vi "Sub Pic Write Data.vi"(8 "error in (no error)":errorcluster, 10 "data (RGB format)":u32[][](array[numeric]) format="%x", 11 "Main Panel in":refnum<class "Main Panel.lvclass">) -> (0 "error out":errorcluster, 3 "Main Panel out":refnum<class "Main Panel.lvclass">)   [LabVIEW 2018, in "Main Panel.lvlib" / "Main Panel.lvclass"]
uses:
  Main Panel.lvclass
  Main Panel.lvclass/Main Panel.ctl
  <vilib>/picture/picture.llb/Draw True-Color Pixmap.vi
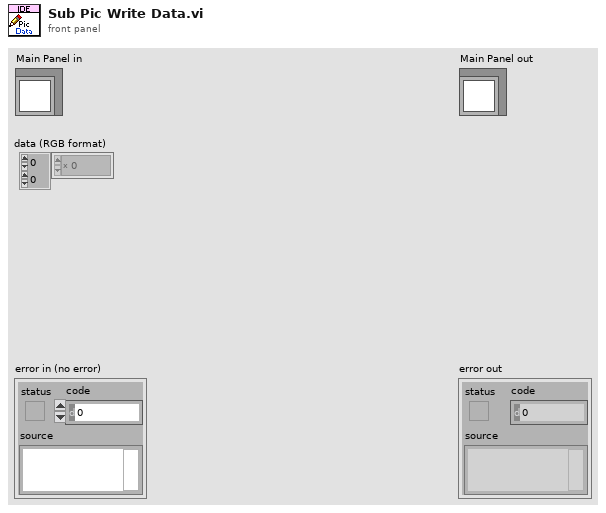
[diagram p1: front panel]
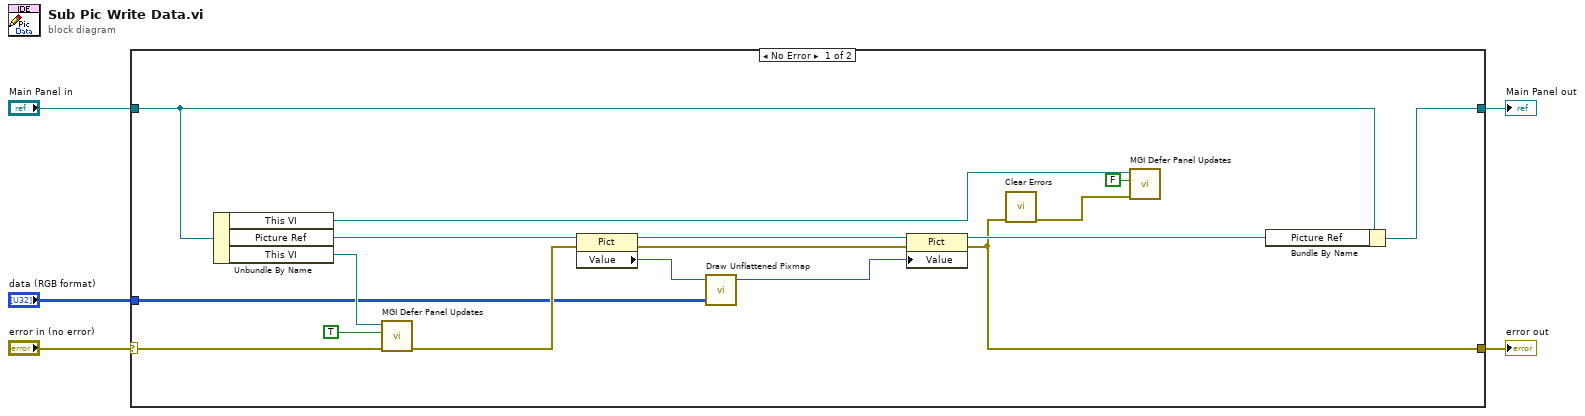
[diagram p0: block diagram]
diagram:
  n1 = case shown="No Error" "error in (no error)" {
    selector: "error in (no error)" -> [w20 w24]
    tunnel: [w6 w24] -> w4
    tunnel: [w11 w23] -> w2
    tunnel: "Main Panel in" -> [w22 w23]
    tunnel: "data (RGB format)" -> [w12 _]
    frame No Error {
      n2 = Unbundle By Name(w22) -> ("This VI"=w8:refnum<vi>, "Picture Ref"=w18:refnum<vi>, "This VI"=w21:refnum<vi>)
      n3 = call <userlib>:"MGI Defer Panel Updates.vi"("Error In"=w20, "Defer Updates?"=TRUE, "VI Reference (Caller)"=w21) -> ("Error Out"=w17:errorcluster)  [unwired: 8 in]
      n4 = property class="Pict"(reference=w18, error in=w17) -> (reference out=w15:refnum<vi>, error out=w14:errorcluster, "Value"=w16:picture)
      n5 = call-poly <vilib>:"Draw Unflattened Pixmap.vi"("picture"=w16, "data (RGB format)"=w12) -> ("new picture"=w13:picture)  [unwired: 7 in]
      n6 = property class="Pict"(reference=w15, error in=w14, "Value"=w13) -> (reference out=w10:refnum<vi>, error out=w6:errorcluster)
      n7 = call <vilib>:"Clear Errors.vi"("error in (no error)"=w6) -> ("error out"=w9:errorcluster)  [unwired: 5 in, 1 out]
      n8 = call <userlib>:"MGI Defer Panel Updates.vi"("Error In"=w9, "Defer Updates?"=FALSE, "VI Reference (Caller)"=w8) -> ()  [unwired: 8 in, 1 out]
      n9 = Bundle By Name(cluster=w22, "Picture Ref"=w10) -> (w11:refnum<class "Main Panel.lvclass">)
    }
    frame Error {
    }
  }
  "error out" <- w4
  "Main Panel out" <- w2
